vi "Initialize.vi"(8 "error in (no error)":errorcluster, 10 "Device":string, 11 "Optical Spectrum Analyzer In":refnum<class "Optical Spectrum Analyzer.lvclass">) -> (0 "error out":errorcluster, 3 "Optical Spectrum Analyzer Out":refnum<class "Optical Spectrum Analyzer.lvclass">)   [LabVIEW 2018, in "Optical Spectrum Analyzer.lvlib" / "Optical Spectrum Analyzer.lvclass"]
uses:
  Optical Spectrum Analyzer.lvclass
  Optical Spectrum Analyzer.lvclass/Optical Spectrum Analyzer.ctl
  PPLs/Configuration/Configuration.lvlibp/Configuration.lvclass
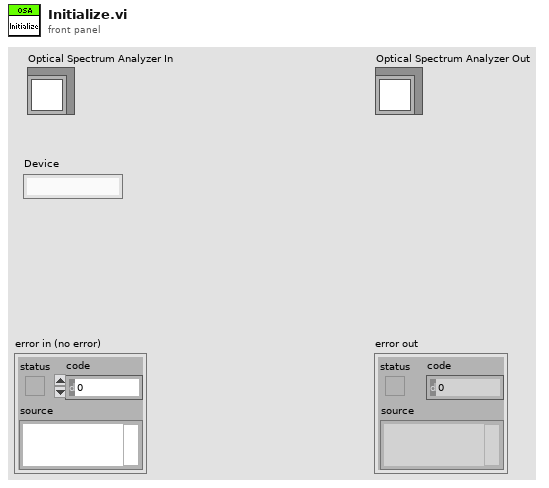
[diagram p1: front panel]
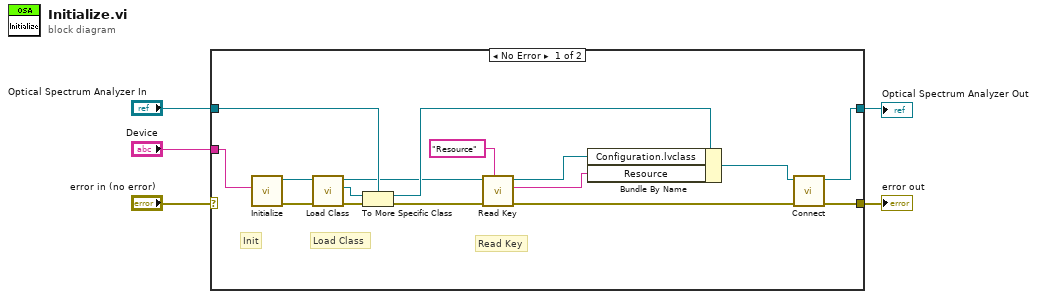
[diagram p0: block diagram]
diagram:
  n1 = case shown="No Error" "error in (no error)" {
    selector: "error in (no error)" -> [_ w23]
    tunnel: [w18 w23] -> w4
    tunnel: "Optical Spectrum Analyzer In" -> [w21 w22]
    tunnel: [w17 w22] -> w2
    tunnel: "Device" -> [w16 _]
    frame No Error {
      # "Read Key"
      # "Load Class"
      # "Init"
      n2 = call "Initialize.vi"("Device"=w16) -> ("error out"=w15:errorcluster, "Configuration out"=w12:refnum<class "Configuration.lvclass">)  [unwired: 9 in]
      n3 = call "Load Class.vi"("error in"=w15, "Configuration in"=w12) -> ("error out"=w14:errorcluster, "Class out"=w13:refnum<class>, "Configuration out"=w7:refnum<class "Configuration.lvclass">)  [unwired: 7 in]
      n4 = To More Specific Class(target class=w21, reference=w13, error in=w14) -> (specific class reference=w20:refnum<class "Optical Spectrum Analyzer.lvclass">, error out=w10:errorcluster)
      n5 = call "Read Key.vi"("Key:"="Resource", "error in"=w10, "Configuration in"=w7) -> ("error out"=w9:errorcluster, "Value"=w8:string, "Configuration out"=w6:refnum<class "Configuration.lvclass">)  [unwired: 6 in]
      n6 = Bundle By Name(cluster=w20, "Configuration.lvclass"=w6, "Resource"=w8) -> (w19:refnum<class "Optical Spectrum Analyzer.lvclass">)
      n7 = call-dynamic "Connect.vi"("error in (no error)"=w9, "Optical Spectrum Analyzer in"=w19) -> ("error out"=w18:errorcluster, "Optical Spectrum Analyzer out"=w17:refnum<class "Optical Spectrum Analyzer.lvclass">)  [unwired: 8 in]
    }
    frame Error {
    }
  }
  "error out" <- w4
  "Optical Spectrum Analyzer Out" <- w2
